vi "Quick Usb Get Dll Version.vi"(8 "error in (no error)":errorcluster, 9 "BuildDllVersion":u16, 10 "MinorDllVersion":u16, 11 "MajorDllVersion":u16) -> (0 "error out":errorcluster, 1 "BuildDllVersion out":u16, 2 "MinorDllVersion out":u16, 3 "MajorDllVersion out":u16, 5 "function return":i32)   [LabVIEW 2011, in "QuickUSB.lvlib"]
doc: "QUSBLIB QRETURN QuickUsbGetDllVersion(\n PQWORD MajorDllVersion,\n PQWORD MinorDllVersion,\n PQWORD BuildDllVersion\n);"
uses:
  QuickUSB.lvlib
  QuickUSB.dll
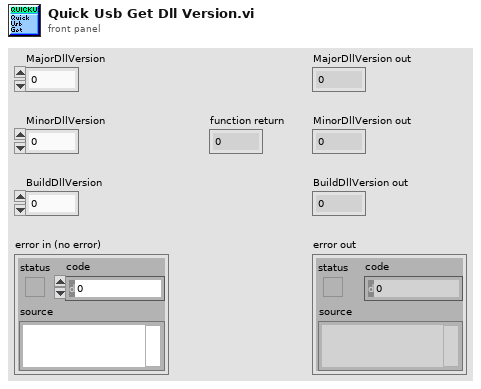
[diagram p1: front panel]
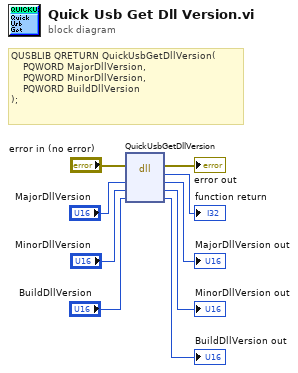
[diagram p0: block diagram]
diagram:
  # "QUSBLIB QRETURN QuickUsbGetDllVersion(\n    PQWORD MajorDllVersion,\n    PQWORD MinorDllVersion,\n    PQWORD BuildDllVersion\n);"
  n1 = dll-call lib="C:/QuickUSB/QuickUSB.*" fn="QuickUsbGetDllVersion"(error in="error in (no error)", "MajorDllVersion"="MajorDllVersion", "MinorDllVersion"="MinorDllVersion", "BuildDllVersion"="BuildDllVersion") -> (error out=→"error out":errorcluster, →"function return":i32, "MajorDllVersion"=→"MajorDllVersion out":u16, "MinorDllVersion"=→"MinorDllVersion out":u16, "BuildDllVersion"=→"BuildDllVersion out":u16)  [unwired: 2 in, 1 out]
